vi "medicaoIXV.vi"() -> ()   [LabVIEW 2012]
uses:
  <vilib>/Utility/file.llb/Write To Spreadsheet File (string).vi
  <vilib>/Utility/file.llb/Write To Spreadsheet File (DBL).vi
  <instrlib>/Agilent 6XXX Series/Agilent 6XXX Series.lvlib
panel:
  out "reset graph":bool=TRUE
  out "array":dbl[][](array[numeric])
  in  "Tab Control":enum32{"Entrada de dados", "Saída de dados"}(tab)
  out "ON/OFF":bool
  in  "Pontos":dbl
  in  "Tensão máxima":dbl
  in  "Nome da célula":string
  in  "Local":path
  in  "Delay(ms)":dbl
  in  "Start":bool
  in  "Print Screen":bool
  out "IXV":cluster{"Y":dbl[], "Y":dbl[]}[](graph)
  out "output voltage":dbl
  out "Tensao Atual":dbl
  out "Corrente Atual":dbl
  out "Ponto Atual":i32
  out "TABELA DE DADOS\nTensão(fonte)     Tensão                  Corrente            Pontos":dbl[][](array[numeric]) caption="all rows" format="%0.3f"
  in  "stop":bool
  in  "CorrenteGraph":dbl
  in  "error in (no error)":errorcluster
  out "error out":errorcluster
  in  "TensaoGraph":dbl
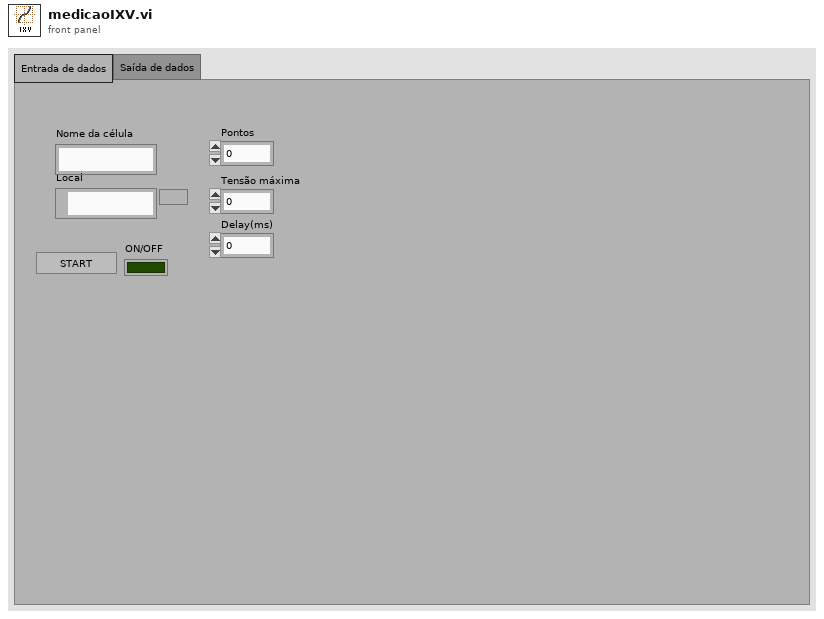
[diagram p1: front panel]
types:
  T1 = typedef "imagedata.ctl" = cluster{"image type":i32, "image depth":i32, "image":u8[], "mask":u8[], "colors":u32[], "Rectangle":cluster{"left":i16, "top":i16, "right":i16, "bottom":i16}}
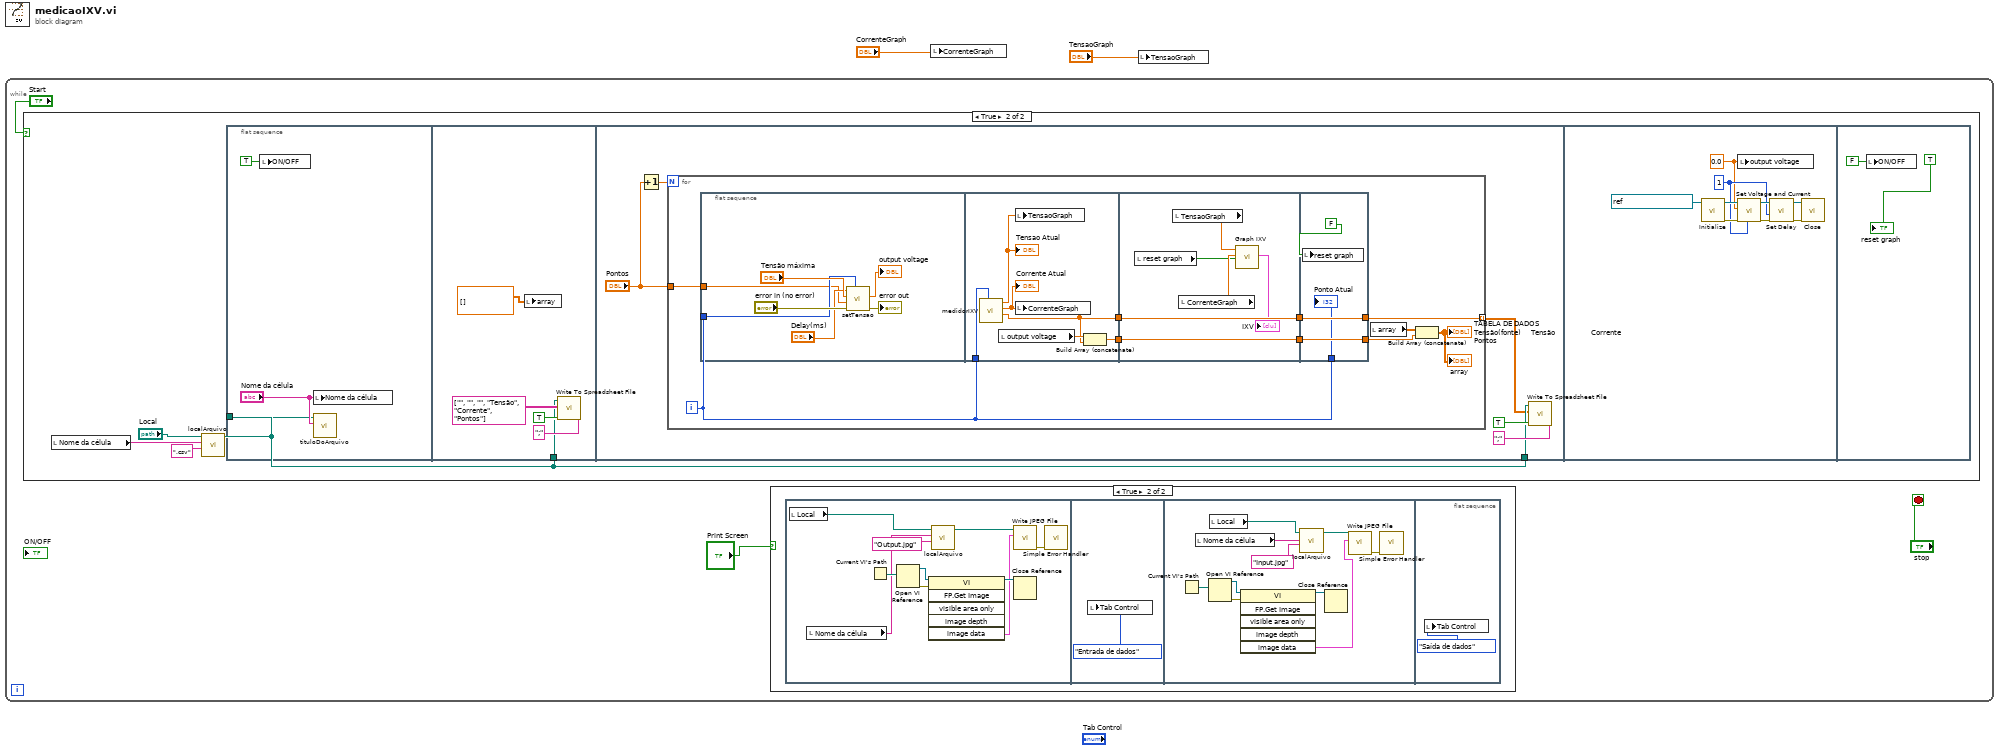
[diagram p0: block diagram]
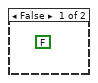
[diagram p3: hidden frame]
diagram:
  n1 = while {
    stop <- "stop" stop-if-true
    n2 = case shown="True" "Start" {
      frame False {
        (unwired) FALSE
      }
      frame True {
        n3 = local read "Nome da célula"() -> (w29:string)
        n4 = call "localArquivo.vi"("extensão"=".csv", "Nome do arquivo"=w29, "Local"="Local") -> ("Path"=w28:path)  [unwired: 8 in]
        n5 = flat-sequence {
          tunnel: w28 -> [w33]
          tunnel: w28 -> [w36]
          tunnel: w28 -> [w43]
          frame #0 {
            n6 = local write "ON/OFF"(TRUE ("ON/OFF")) -> ()
            n7 = local write "Nome da célula"("Nome da célula") -> ()
            n8 = call "tituloDoArquivo.vi"("Nome da célula"="Nome da célula", "file path (dialog if empty)"=w33) -> ()  [unwired: 10 in]
          }
          frame #1 {
            n9 = local write "array"(dbl[][] [] ("array")) -> ()
            n10 = call-poly <vilib>:"Write To Spreadsheet File.vi"("delimiter (\\t)"=";" ("delimiter (\\t)"), "append to file? (new file:F)"=TRUE, "2D data"=string[][] [["", "", ""], ["Tensão", "Corrente", "Pontos"]], "file path (dialog if empty)"=w36) -> ()  [unwired: 4 in, 1 out]
          }
          frame #2 {
            n11 = Increment(x="Pontos") -> (x+1=w42:dbl)
            n12 = for {
              N: w42 -> [_]
              tunnel: [w54] -> w40 mode=indexing
              tunnel: "Pontos" -> [w55]
              i -> [w46]
              n13 = flat-sequence {
                tunnel: w55 -> [w58]
                tunnel: w46 -> [w59]
                tunnel: w46 -> [w68]
                tunnel: [w63] -> w53
                tunnel: [w65] -> w52
                tunnel: w53 -> [w74]
                tunnel: w52 -> [w73]
                tunnel: [w74] -> w48
                tunnel: [w73] -> w47
                tunnel: [w77] -> w51
                tunnel: [w78] -> w54
                tunnel: w48 -> [w78]
                tunnel: w47 -> [w77]
                tunnel: w46 -> [w76]
                frame #0 {
                  n14 = call "setTensao.vi"("Ponto"=w59, "error in (no error)"="error in (no error)", "Pontos"=w58, "Tensão máxima"="Tensão máxima", "delay(ms)"="Delay(ms)") -> ("error out"=→"error out":errorcluster, "output voltage"=→"output voltage":dbl)  [unwired: 5 in]
                }
                frame #1 {
                  n15 = call "medidorIXV.vi"("Ponto"=w68) -> ("Array"=w63:dbl[], "Corrente Atual"=w67:dbl, "Tensao Atual"=w66:dbl)  [unwired: 8 in]
                  "Corrente Atual" <- w67
                  "Tensao Atual" <- w66
                  n16 = local read "output voltage"() -> (w64:dbl)
                  n17 = local write "TensaoGraph"(w66) -> ()
                  n18 = local write "CorrenteGraph"(w67) -> ()
                  n19 = Build Array (concatenate)(w64, w63) -> (w65:dbl[])
                }
                frame #2 {
                  n20 = local read "reset graph"() -> (w69:bool)
                  n21 = local read "TensaoGraph"() -> (w72:dbl)
                  n22 = local read "CorrenteGraph"() -> (w71:dbl)
                  n23 = call "Graph IXV"("Reset"=w69, "Y Input"=w71, "X Input"=w72) -> ("XY Graph"=→"IXV":cluster{"Y":dbl[], "Y":dbl[]}[])  [unwired: 2 in, 6 out]
                }
                frame #3 {
                  n24 = local write "reset graph"(FALSE) -> ()
                  "Ponto Atual" <- w76
                }
              }
              n25 = local read "array"() -> (w50:dbl[][])
              n26 = Build Array (concatenate)(w50, w51) -> (→"TABELA DE DADOS\nTensão(fonte)     Tensão                  Corrente            Pontos" →"array":dbl[][])
            }
            n27 = call-poly <vilib>:"Write To Spreadsheet File.vi"("delimiter (\\t)"=";" ("delimiter (\\t)"), "append to file? (new file:F)"=TRUE, "2D data"=w40, "file path (dialog if empty)"=w43) -> ()  [unwired: 4 in, 1 out]
          }
          frame #3 {
            w79 = 0.0 ("voltage (0 V)")
            w82 = u8 1 ("channel (1)")
            n28 = call <instrlib>:"Initialize.vi"("VISA resource name"=refnum<visa-resource-name> "GPIB0::5::INSTR") -> ("error out"=w84:errorcluster, "VISA resource name out"=w83:refnum<visa-resource-name>)  [unwired: 9 in]
            n29 = local write "output voltage"(w79) -> ()
            n30 = call <instrlib>:"Set Voltage and Current.vi"("channel (1)"=w82, "error in (no error)"=w84, "voltage (0 V)"=w79, "VISA resource name"=w83) -> ("error out"=w85:errorcluster, "VISA resource name out"=w86:refnum<visa-resource-name>)  [unwired: 6 in]
            n31 = call <instrlib>:"Set Delay.vi"("error in (no error)"=w85, "channel (1)"=w82, "VISA resource name"=w86) -> ("error out"=w80:errorcluster, "VISA resource name out"=w81:refnum<visa-resource-name>)  [unwired: 7 in]
            n32 = call <instrlib>:"Close.vi"("error in (no error)"=w80, "VISA resource name"=w81) -> ()  [unwired: 9 in, 1 out]
          }
          frame #4 {
            n33 = local write "ON/OFF"(FALSE) -> ()
            "reset graph" <- TRUE
          }
        }
      }
    }
    n34 = case shown="True" "Print Screen" {
      frame False {
      }
      frame True {
        n35 = flat-sequence {
          frame #0 {
            n36 = local read "Local"() -> (w7:path)
            n37 = local read "Nome da célula"() -> (w6:string)
            n38 = Current VI's Path() -> (path=w12:path)
            n39 = Open VI Reference(vi path=w12) -> (vi reference=w13:refnum<vi>, error out=w14:errorcluster)  [unwired: 5 in]
            n40 = invoke class="VI" method="FP.Get Image"(reference=w13, error in=w14) -> (reference out=w11:refnum<vi>, "image data"=w10:T1)  [unwired: 4 in, 4 out]
            n41 = call "localArquivo.vi"("extensão"="Output.jpg", "Nome do arquivo"=w6, "Local"=w7) -> ("Path"=w15:path)  [unwired: 8 in]
            n42 = call <vilib>:"Write JPEG File.vi"("image data"=w10, "path to JPEG file"=w15) -> ("error out"=w9:errorcluster)  [unwired: 8 in, 1 out]
            n43 = Close Reference(reference=w11) -> ()  [unwired: 1 in, 1 out]
            n44 = call <vilib>:"Simple Error Handler.vi"("error in (no error)"=w9) -> ()  [unwired: 4 in, 5 out]
          }
          frame #1 {
            n45 = local write "Tab Control"(enum32{"Entrada de dados", "Saída de dados"}."Entrada de dados" ("Tab Control")) -> ()
          }
          frame #2 {
            n46 = Current VI's Path() -> (path=w25:path)
            n47 = local read "Nome da célula"() -> (w18:string)
            n48 = Open VI Reference(vi path=w25) -> (vi reference=w24:refnum<vi>, error out=w23:errorcluster)  [unwired: 5 in]
            n49 = local read "Local"() -> (w17:path)
            n50 = invoke class="VI" method="FP.Get Image"(reference=w24, error in=w23) -> (reference out=w26:refnum<vi>, "image data"=w21:T1)  [unwired: 4 in, 4 out]
            n51 = call "localArquivo.vi"("extensão"="Input.jpg", "Nome do arquivo"=w18, "Local"=w17) -> ("Path"=w20:path)  [unwired: 8 in]
            n52 = Close Reference(reference=w26) -> ()  [unwired: 1 in, 1 out]
            n53 = call <vilib>:"Write JPEG File.vi"("image data"=w21, "path to JPEG file"=w20) -> ("error out"=w22:errorcluster)  [unwired: 8 in, 1 out]
            n54 = call <vilib>:"Simple Error Handler.vi"("error in (no error)"=w22) -> ()  [unwired: 4 in, 5 out]
          }
          frame #3 {
            n55 = local write "Tab Control"(enum32{"Entrada de dados", "Saída de dados"}."Saída de dados" ("Tab Control")) -> ()
          }
        }
      }
    }
  }
  n56 = local write "CorrenteGraph"("CorrenteGraph") -> ()
  n57 = local write "TensaoGraph"("TensaoGraph") -> ()
